vi "Query Trace Data.vi"(8 "error in (no error)":errorcluster, 10 "Trace Number":u8=1, 11 "VNA-CMT S2 S4 in":refnum<class "VNA-CMT S2 S4.lvclass">) -> (0 "error out":errorcluster, 1 "Data":dbl[](array[numeric]), 2 "Frequency":dbl[](array[numeric]), 3 "VNA-CMT S2 S4 out":refnum<class "VNA-CMT S2 S4.lvclass">)   [LabVIEW 2020, in "VNA-CMT S2 S4.lvclass"]
doc: "Query the active trace data.\nIt returns both x and y data"
uses:
  VNA-CMT S2 S4.lvclass
  C:/Sandbox/Git_Sandbox/WiSpry Test Framework source code (LV20)/WiSpry Test Framework/Instruments/Instrument.lvclass
  Instrument.lvclass/Instrument.ctl
  Instrument.lvclass
  <instrlib>/CMT S2 and S4 VNA/CMT S2 and S4 VNA.lvlib
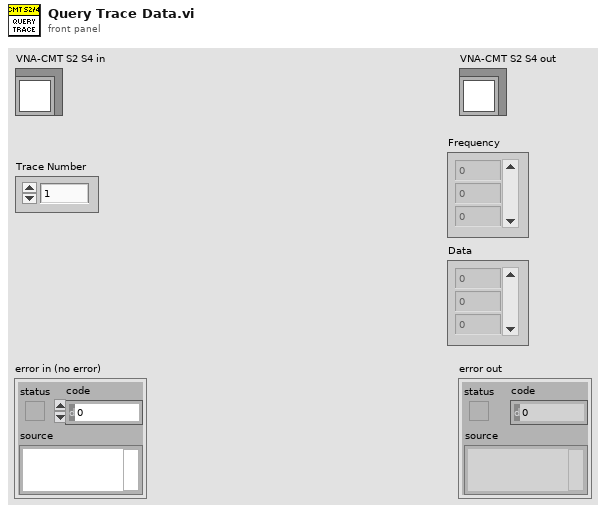
[diagram p1: front panel]
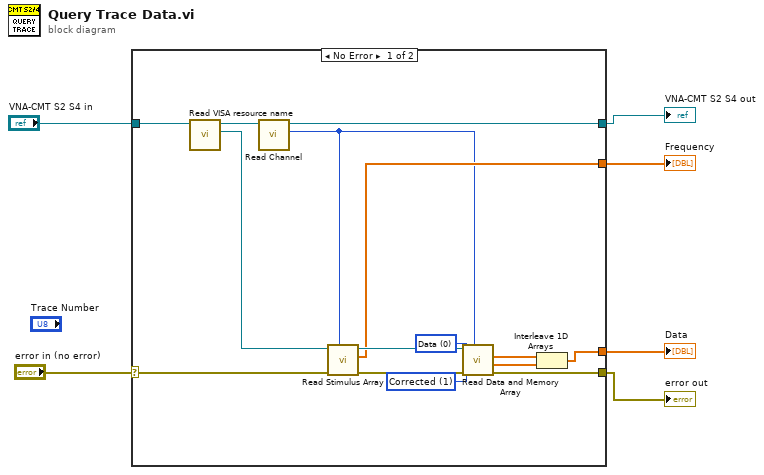
[diagram p0: block diagram]
diagram:
  n1 = case shown="No Error" "error in (no error)" {
    selector: "error in (no error)" -> [w16 w23]
    tunnel: [w20 w23] -> w3
    tunnel: [w8 w22] -> w4
    tunnel: "VNA-CMT S2 S4 in" -> [w21 w22]
    tunnel: [w10 _] -> w2
    tunnel: [w15 _] -> w1
    frame No Error {
      w13 = u16 0 items=["Data", "Memory"] ("Source (0: Data)")
      w14 = u16 1 items=["Formatted", "Corrected"] ("Correction (0: Data)")
      n2 = call "Read VISA resource name.vi"("Instrument in"=w21) -> ("VISA resource name"=w19:refnum<visa-resource-name>, "Instrument out"=w9:refnum<class "VNA-CMT S2 S4.lvclass">)  [unwired: 9 in]
      n3 = call-dynamic "Read Channel.vi"("Vector Network Analyzer in"=w9) -> ("Channel"=w7:i32, "Vector Network Analyzer out"=w8:refnum<class "VNA-CMT S2 S4.lvclass">)  [unwired: 9 in]
      n4 = call <instrlib>:"Read Stimulus Array.vi"("Channel (1)"=w7, "error in (no error)"=w16, "VISA resource name"=w19) -> ("error out"=w17:errorcluster, "Stimulus Data"=w15:dbl[], "VISA resource name out"=w18:refnum<visa-resource-name>)  [unwired: 6 in]
      n5 = call <instrlib>:"Read Data and Memory Array.vi"("Channel (1)"=w7, "error in (no error)"=w17, "Correction (0: Data)"=w14, "Source (0: Data)"=w13, "VISA resource name"=w18) -> ("error out"=w20:errorcluster, "Secondary / Imaginary"=w11:dbl[], "Primary / Real"=w12:dbl[])  [unwired: 3 in, 1 out]
      n6 = Interleave 1D Arrays(w12, w11) -> (w10:dbl[])
    }
    frame Error {
    }
  }
  "error out" <- w3
  "VNA-CMT S2 S4 out" <- w4
  "Data" <- w2
  "Frequency" <- w1
